vi "View.vi"(8 "error in (no error)":errorcluster, 10 "Debugger":refnum<class "Debug Process.lvclass">, 11 "List View In":refnum<class "Multicolumn List Box View.lvclass">) -> (0 "error out":errorcluster)   [LabVIEW 2020, in "Multicolumn List Box View.lvclass"]
uses:
  Multicolumn List Box View.lvclass
  C:/Users/anton/Documents/GitHub/triarc-debugger/source/Debug View/Debug View.lvclass
  Process/Debug Process.lvclass
  Process/Debug Process.lvclass/Debug Process.ctl
  Debug View/Debug View.lvclass/Debug View.ctl
  Multicolumn List Box View.lvclass/Multicolumn List Box View.ctl
  <vilib>/Utility/miscctls.llb/LVRowAndColumnUnsignedTypeDef.ctl
  Debugger/Debugger.lvclass
  <vilib>/Utility/miscctls.llb/LVRowAndColumnTypeDef.ctl
  Multicolumn List Box View Model/Multicolumn List Box View Model.lvclass
  Debug View/Debug View.lvclass
panel:
  in  "Multicolumn Listbox":i32(listbox) caption="Listbox"
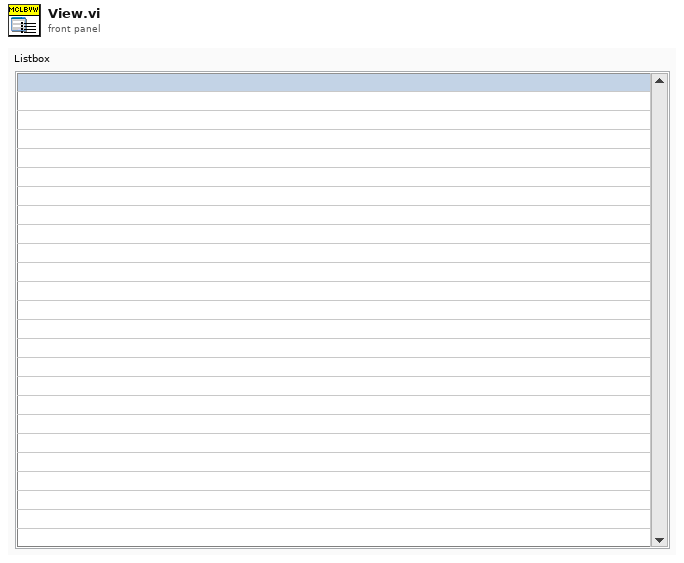
[diagram p1: front panel]
types:
  T1 = typedef "LVRowAndColumnUnsignedTypeDef.ctl" = cluster{"Row":u32, "Column":u32}
  T2 = typedef "LVRowAndColumnTypeDef.ctl" = cluster{"Row":i32, "Column":i32}
  T3 = typedef "LVRectTypeDef.ctl" = cluster{"Left":i16, "Top":i16, "Right":i16, "Bottom":i16}
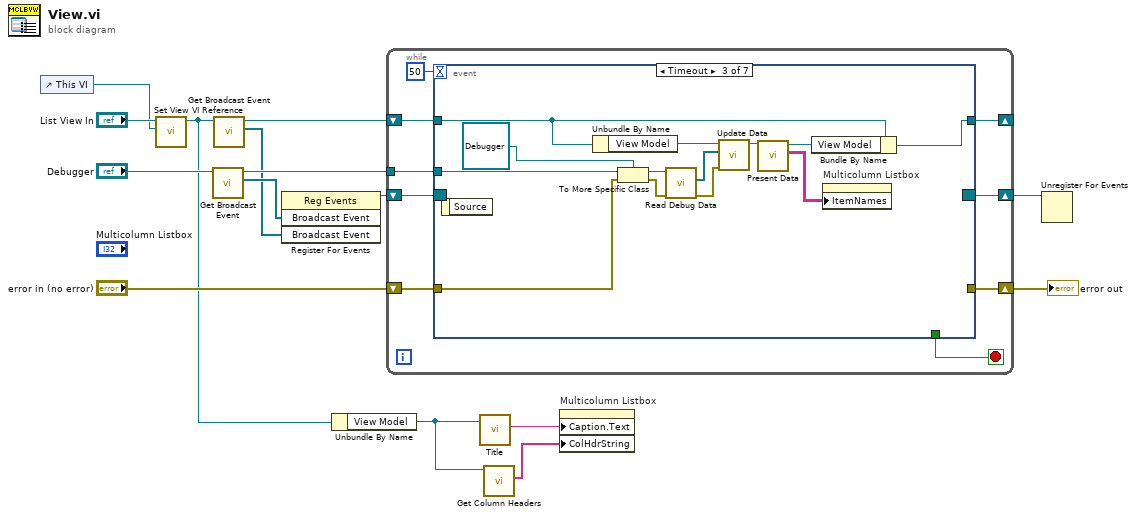
[diagram p0: block diagram]
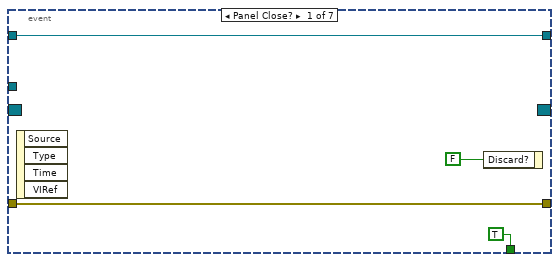
[diagram p2: hidden frame]
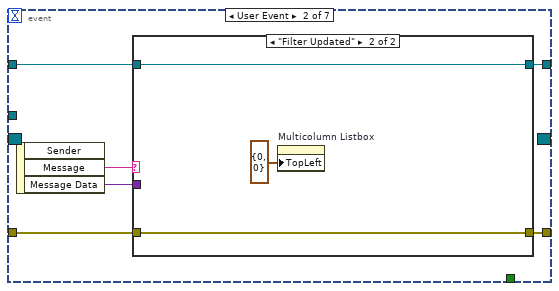
[diagram p3: hidden frame]
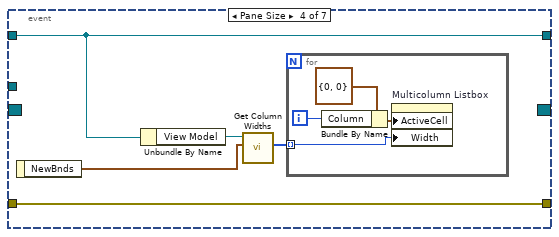
[diagram p5: hidden frame]
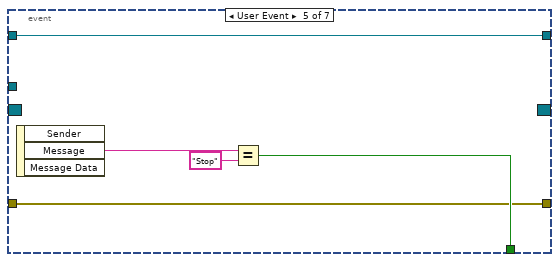
[diagram p6: hidden frame]
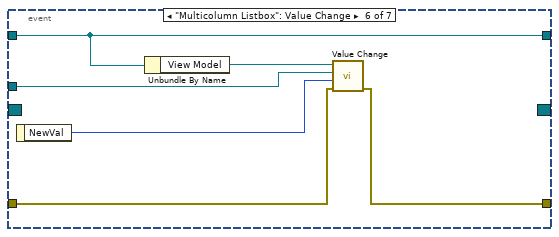
[diagram p7: hidden frame]
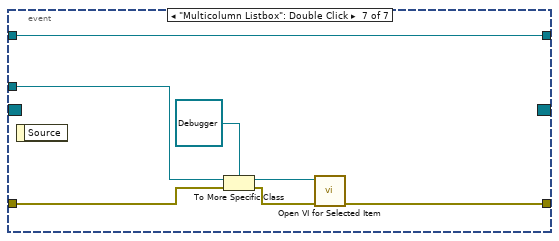
[diagram p8: hidden frame]
diagram:
  n1 = control-ref of="This VI"() -> (w3:refnum<vi>)
  n2 = call "Set View VI Reference.vi"("View VI ref"=w3, "Debug View in"="List View In") -> ("Debug View out"=w4:refnum<class "Multicolumn List Box View.lvclass">)  [unwired: 8 in, 1 out]
  n3 = call "Get Broadcast Event.vi"("Process in"="Debugger") -> ("Broadcast Event"=w8:refnum<user-event>[], "Process out"=w10:refnum<class "Debug Process.lvclass">)  [unwired: 8 in, 1 out]
  n4 = call "Get Broadcast Event.vi"("Debug View In"=w4) -> ("Broadcast Event"=w5:refnum<user-event>[], "Debug View Out"=w6:refnum<class "Multicolumn List Box View.lvclass">)  [unwired: 8 in, 1 out]
  n5 = register-events(w8, w5) -> (reference out=w9:refnum<event-registration>)  [unwired: 2 in, 1 out]
  n6 = Unbundle By Name(w4) -> ("View Model"=w2:refnum<class "Multicolumn List Box View Model.lvclass">)
  n7 = while {
    shift-right: [w23] -> _
    shift-left: w6 -> [w24]
    shift-right: [w22] -> w15
    shift-left: "error in (no error)" -> [w21]
    shift-right: [w20] -> w13
    shift-left: w9 -> [w19]
    tunnel: w10 -> [w18]
    stop <- w17 stop-if-true
    n8 = event shown="[2] Timeout" {
      selector: w19 -> [_ _ _ _ _ _ _]
      dyn-events: [_ _ _ _ _ _ _] -> w20
      timeout: 50 -> [_ _ _ _ _ _ _]
      tunnel: w24 -> [w28 w30 w48 w57 w62 w72 w74]
      tunnel: [w28 w29 w47 w57 w62 w72 w74] -> w23
      tunnel: [w27 w33 _ w53 w63 w69 w73] -> w22
      tunnel: w21 -> [w27 w32 w40 w53 w63 w68 w75]
      tunnel: w18 -> [_ _ w46 _ _ w70 w76]
      tunnel: [TRUE ("Discard?") _ _ _ w64 _ _] -> w17
      event Panel Close? {
        n9 = event-data() -> ()  [unwired: 1 in, 4 out]
        n10 = event-data("Discard?"=FALSE) -> ()  [unwired: 1 in, 1 out]
      }
      event User Event {
        n11 = event-data() -> ("Message"=w34:string, "Message Data"=w31:variant)  [unwired: 1 in, 1 out]
        n12 = case shown="\"Filter Updated\"" w34 {
          tunnel: [w36 w38] -> w33
          tunnel: w32 -> [w36 w38]
          tunnel: w31 -> [_ _]
          tunnel: w30 -> [w35 w39]
          tunnel: [w35 w39] -> w29
          frame Default {
          }
          frame "Filter Updated" {
            n13 = property on="Multicolumn Listbox" class="MCListbox (strict)"("TopLeft"=T1 {"Row"=0, "Column"=0} ("Top Left Visible Cell")) -> ()  [unwired: 2 in, 2 out]
          }
        }
      }
      event Timeout {
        n14 = event-data() -> ()  [unwired: 1 in, 1 out]
        n15 = Unbundle By Name(w48) -> ("View Model"=w52:refnum<class "Multicolumn List Box View Model.lvclass">)
        n16 = To More Specific Class(target class=refnum<class "Debugger.lvclass"> refnum ("Debugger Out"), reference=w46, error in=w40) -> (specific class reference=w45:refnum<class "Debugger.lvclass">, error out=w42:errorcluster)
        n17 = call "Read Debug Data.vi"("error in (no error)"=w42, "Debugger In"=w45) -> ("error out"=w41:errorcluster, "Data Log"=w43:refnum<class "Debug Data.lvclass">[])  [unwired: 7 in, 1 out]
        n18 = call-dynamic "Update Data.vi"("error in (no error)"=w41, "Debug Data"=w43, "List Seen Processes View Model In"=w52) -> ("List Seen Processes View Model Out"=w49:refnum<class "Multicolumn List Box View Model.lvclass">)  [unwired: 7 in, 1 out]
        n19 = call "Present Data.vi"("List Seen Processes View Model In"=w49) -> ("Data"=w51:string[][], "List Seen Processes View Model Out"=w50:refnum<class "Multicolumn List Box View Model.lvclass">)  [unwired: 8 in, 1 out]
        n20 = Bundle By Name(cluster=w48, "View Model"=w50) -> (w47:refnum<class "Multicolumn List Box View.lvclass">)
        n21 = property on="Multicolumn Listbox" class="MCListbox (strict)"("ItemNames"=w51) -> ()  [unwired: 2 in, 2 out]
      }
      event Pane Size {
        n22 = event-data() -> ("NewBnds"=w54:T3)  [unwired: 1 in]
        n23 = Unbundle By Name(w57) -> ("View Model"=w56:refnum<class "Multicolumn List Box View Model.lvclass">)
        n24 = call "Get Column Widths.vi"("NewBnds"=w54, "Multicolumn List Box View Model In"=w56) -> ("Widths"=w55:i32[])  [unwired: 7 in, 2 out]
        n25 = for {
          tunnel: w55 -> [w58] mode=indexing
          i -> [w59]
          n26 = Bundle By Name(cluster=T2 {"Row"=0, "Column"=0} ("Active Cell:Active Cell"), "Column"=w59) -> (w60:T2)
          n27 = property on="Multicolumn Listbox" class="MCListbox (strict)"("ActiveCell"=w60, "Width"=w58) -> ()  [unwired: 2 in, 2 out]
        }
      }
      event User Event {
        n28 = event-data() -> ("Message"=w66:string)  [unwired: 1 in, 2 out]
        n29 = Equal?(x=w66, y="Stop") -> (x = y?=w64:bool)
      }
      event "Multicolumn Listbox": Value Change {
        n30 = event-data() -> ("NewVal"=w67:i32)  [unwired: 1 in]
        n31 = Unbundle By Name(w72) -> ("View Model"=w71:refnum<class "Multicolumn List Box View Model.lvclass">)
        n32 = call-dynamic "Value Change.vi"("error in (no error)"=w68, "NewVal"=w67, "Debugger"=w70, "List Box View Model In"=w71) -> ("error out"=w69:errorcluster)  [unwired: 6 in, 1 out]
      }
      event "Multicolumn Listbox": Double Click {
        n33 = event-data() -> ()  [unwired: 1 in, 1 out]
        n34 = To More Specific Class(target class=refnum<class "Debugger.lvclass"> refnum ("Debugger.lvclass"), reference=w76, error in=w75) -> (specific class reference=w78:refnum<class "Debugger.lvclass">, error out=w77:errorcluster)
        n35 = call "Open VI for Selected Item.vi"("error in (no error)"=w77, "Debugger In"=w78) -> ("error out"=w73:errorcluster)  [unwired: 8 in, 1 out]
      }
    }
  }
  "error out" <- w15
  n36 = call-dynamic "Title.vi"("List Box View Model in"=w2) -> ("Title"=w12:string)  [unwired: 8 in, 2 out]
  n37 = call "Get Column Headers.vi"("Multicolumn List Box View Model In"=w2) -> ("Header Strings"=w1:string[])  [unwired: 8 in, 2 out]
  n38 = property on="Multicolumn Listbox" class="MCListbox (strict)"("Caption.Text"=w12, "ColHdrString"=w1) -> ()  [unwired: 2 in, 2 out]
  n39 = Unregister For Events(event registration refnum=w13) -> ()  [unwired: 1 in, 1 out]
